vi "Build Command.vi"(8 "error in (no error)":errorcluster, 11 "Executable in":refnum<class "Executable.lvclass">) -> (0 "error out":errorcluster, 2 "Command":string, 3 "Executable out":refnum<class "Executable.lvclass">)   [LabVIEW 2023, in "HAF.lvlib" / "Executable.lvclass"]
doc: "Builds a command string up for execution on the Instrument by the Driver.  The command consists of a Base command plus any parameters that should be applied."
uses:
  Executable.lvclass
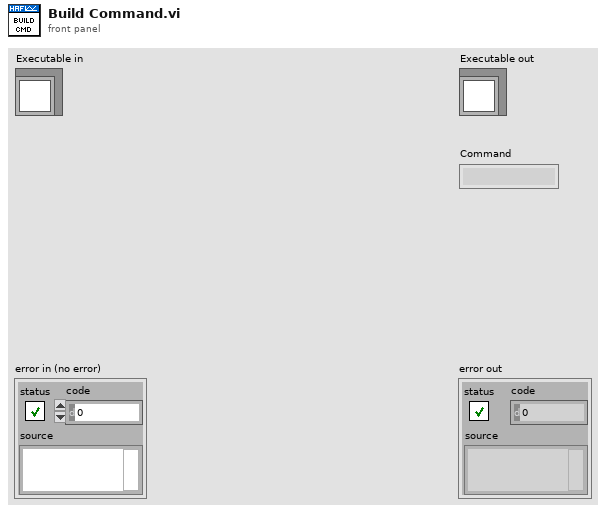
[diagram p1: front panel]
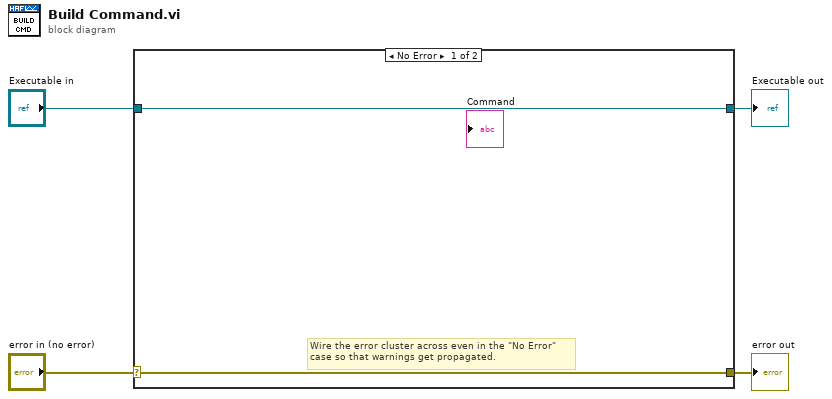
[diagram p0: block diagram]
diagram:
  n1 = case shown="No Error" "error in (no error)" {
    selector: "error in (no error)" -> [w5 w8]
    tunnel: [w5 w8] -> w3
    tunnel: [w6 w7] -> w1
    tunnel: "Executable in" -> [w6 w7]
    frame No Error {
      # "Wire the error cluster across even in the \"No Error\"\ncase so that warnings get propagated."
    }
    frame Error {
    }
  }
  "error out" <- w3
  "Executable out" <- w1
